vi "GetLVExplicitMessage.vi"(8 "error in (no error)":errorcluster, 10 "Motor Controller Parameter":T2, 11 "Session in":T1="Default") -> (0 "error out":errorcluster, 1 "GetAttributeSingle":u8[](array[numeric]), 3 "Session out":T1, 4 "Data (U32)":u32)   [LabVIEW 2022 SP3, in "Motor Controller.lvclass"]
uses:
  Motor Controller.lvclass
  Typedefs/Motor Controller Parameter-Get.ctl
  <vilib>/ethernetip/ethernetip.llb/ethernetip.ctl
  <vilib>/ethernetip/ethernetip.lvlib
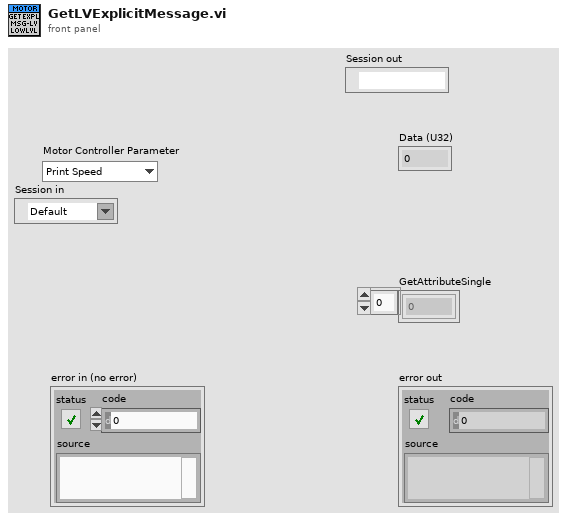
[diagram p1: front panel]
types:
  T1 = typedef "ethernetip.lvlib/ethernetip.ctl" = refnum<k21>
  T2 = typedef "Motor Controller.lvclass/Motor Controller Parameter-Get.ctl" = enum16{"Print Speed", "Jog Speed", "PR Path", "Servo Enabled?", "AlarmCodes"}
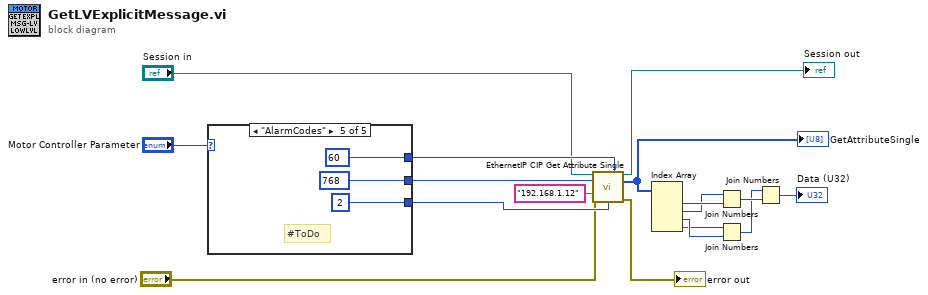
[diagram p0: block diagram]
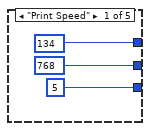
[diagram p2: hidden frame]
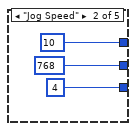
[diagram p3: hidden frame]
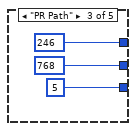
[diagram p4: hidden frame]
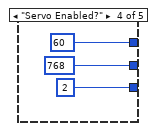
[diagram p5: hidden frame]
diagram:
  n1 = case shown="\"AlarmCodes\"" "Motor Controller Parameter" {
    tunnel: [134 ("Attribute") 10 ("Attribute") 246 ("Attribute") 60 ("Attribute") 60 ("Attribute")] -> w7
    tunnel: [768 ("Class") 768 ("Class") 768 ("Class") 768 ("Class") 768 ("Class")] -> w9
    tunnel: [u32 5 ("assembly instance ID") u32 4 ("assembly instance ID") u32 5 ("assembly instance ID") u32 2 ("assembly instance ID") u32 2 ("assembly instance ID")] -> w8
    frame "Print Speed" {
    }
    frame "Jog Speed" {
    }
    frame "PR Path" {
    }
    frame "Servo Enabled?" {
    }
    frame "AlarmCodes" {
      # "#ToDo"
    }
  }
  n2 = call <vilib>:"EthernetIP CIP Get Attribute Single.vi"("Session in"="Session in", "Network Path"="192.168.1.12", "error in"="error in (no error)", "Class"=w9, "Instance"=w8, "Attribute"=w7) -> ("Session out"=→"Session out":T1, "Data"=w5:u8[], "error out"=→"error out":errorcluster)  [unwired: 7 in]
  "GetAttributeSingle" <- w5
  n3 = Index Array(array=w5) -> (element #1=w16:u8, element #2=w15:u8, element #3=w14:u8, element #4=w13:u8)  [unwired: 4 in]
  n4 = Join Numbers(hi=w15, lo=w16) -> ((hi.lo)=w12:u16)
  n5 = Join Numbers(hi=w13, lo=w14) -> ((hi.lo)=w11:u16)
  n6 = Join Numbers(hi=w11, lo=w12) -> ((hi.lo)=→"Data (U32)":u32)
